vi "Within Range.vi"(8 "error in (no error)":errorcluster, 10 "Range to compare to":refnum<class "Range.lvclass">, 11 "Range in":refnum<class "Range.lvclass">) -> (0 "error out":errorcluster, 1 "Offset":u64, 2 "In Range?":bool, 3 "Range out":refnum<class "Range.lvclass">)   [LabVIEW 2020, in "Range.lvclass"]
uses:
  Range.lvclass
  Range.lvclass/Range.ctl
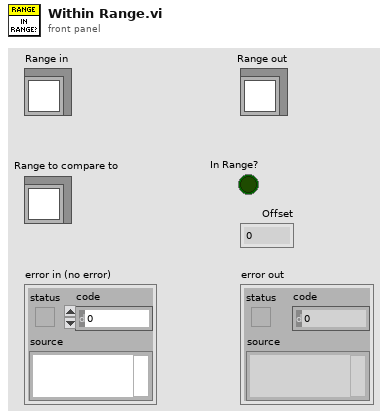
[diagram p1: front panel]
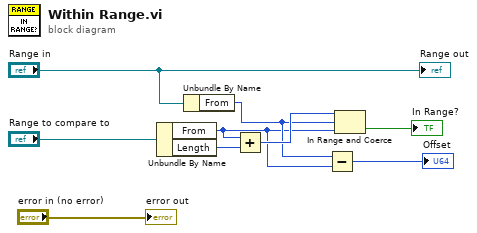
[diagram p0: block diagram]
diagram:
  n1 = Unbundle By Name("Range to compare to") -> ("From"=w2:u64, "Length"=w8:u64)
  n2 = Unbundle By Name("Range in") -> ("From"=w3:u64)
  n3 = Add(x=w2, y=w8) -> (x+y=w7:u64)
  n4 = Subtract(x=w3, y=w2) -> (x-y=→"Offset":u64)
  n5 = In Range and Coerce(upper limit=w7, x=w3, lower limit=w2) -> (In Range?=→"In Range?":bool)  [unwired: 1 out]
  "error out" <- "error in (no error)"
  "Range out" <- "Range in"
